vi "PV Miscellaneous.vi"(8 "error in (no error)":errorcluster, 9 "PV Miscellaneous - Cluster":T1={"Parameter"=0, "Parameter\nread only<->describe"=FALSE, "off<->on   "=TRUE, "Unit adress"=1, "Configuration AO1 (old version)"=0, "Contens of service\nline; # of the 2nd\n parameter"=795, "Configuration DO1 (old version)"=0} {"Configuration DO1 (old version)" items=[" switchpoint attained", " no error", " error", " warning", " error and/or warning", " set speed attained", " pump is on", " accelerates", " decelerater", " always off", " always on", " access request remote"]; "Contens of service\nline; # of the 2nd\n parameter" min=0 max=999 step=1; "Configuration AO1 (old version)" items=[" speed", " power", " current", " lowest value", " highest value"]; "Unit adress" min=1 max=255 step=1; "Parameter" items=[" Preselection brake", " Configuration DO1 (old version)", " Remote operations mode", " Configuration output K4 (old version)", " Configuration AO1 (old version)", " Actual error code (read only)", " Software version electronic drive unit  (read only)", " Software version display and control unit  (read only)", " Parameter set", " Contens of service line (TCM 1601 only)", " Unit adress", " Unit type electronic drive unit", " Error acknowledgement (write only)", " Keyboard interlock (008)", " Seal gas enable (050)"]}, 10 "Adress of unit":u16=1 max=999 step=1, 11 "VISA session":refnum<visa-resource-name>) -> (0 "error out":errorcluster, 2 "response (data)":string, 3 "dup VISA session":refnum<visa-resource-name>)   [LabVIEW 2016, in "Pfeiffer Vacuum.lvlib"]
doc: "There are 15 parameters available, only one of which can be enabled at a time. \n\nPreselection brake (default) (013)\nConfiguration DO1 (024)\n(old version - new in PV Config A D input output)\nRemote operations mode (028)\nConfiguration output K4 (032)\n (old version - new in PV Config A D input output)\nConfiguration AO1 (055)\n (old version - new in PV Config A D input output)\nActual error code (read only) (303)\nSoftware version electronic drive unit (read only) (312)\nSoftware version display and control unit (read only) (351)\nParameter set (794)\nContens of service line (TCM 1601 only) (795)\nUnit adress (797)\nUnit type electronic drive unit (349)\nError acknowledgement (write only) (009)\nKeyboard interlock (008)\nSeal gas enable (050)\n\nNote: Any settings for an parameter that is not selected will be ignored. If a value is out of range, it will be changed to either the upper or the lower limit of the range."
uses:
  Pfeiffer Vacuum.lvlib
  PV Miscellaneous - Cluster.ctl
panel:
  # "Preselection brake             :  \n Remote operations mode  : \n Configuration output K4    : \n Parameter set                      :\n Seal gas enable                   :\n Keyboard interlock            :"
  # "<--------------\n  off\n  stand. operations \n  heat/TMS\n  basic  \n  off\n  off"
  # "----------->          \non \nremote priority \nPWM-signal \n extended \non \non"
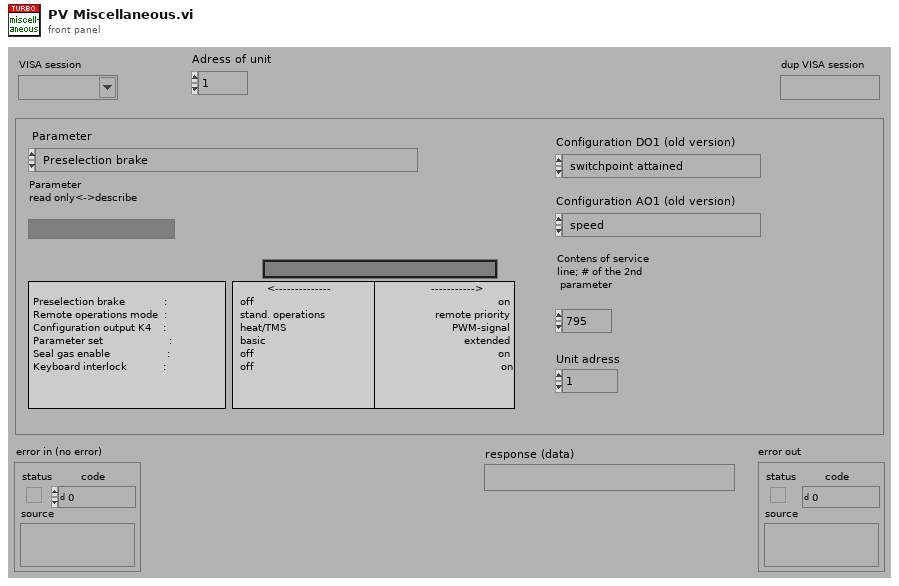
[diagram p1: front panel]
types:
  T1 = typedef "Pfeiffer Vacuum.lvlib/PV Miscellaneous - Cluster.ctl" = cluster{"Parameter":u16, "Parameter\nread only<->describe":bool, "off<->on   ":bool, "Unit adress":i16, "Configuration AO1 (old version)":u16, "Contens of service\nline; # of the 2nd\n parameter":i16, "Configuration DO1 (old version)":u16}
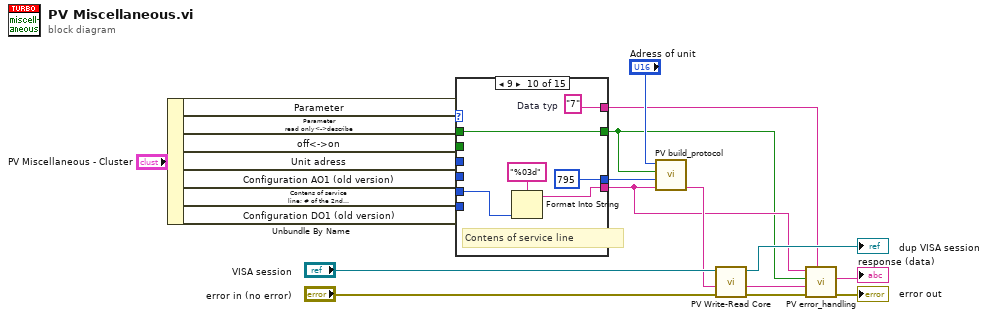
[diagram p0: block diagram]
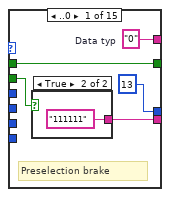
[diagram p2: hidden frame]
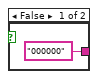
[diagram p3: hidden frame]
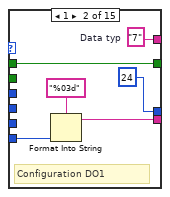
[diagram p4: hidden frame]
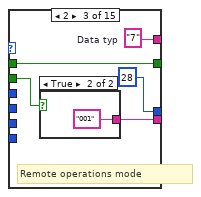
[diagram p5: hidden frame]
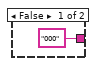
[diagram p6: hidden frame]
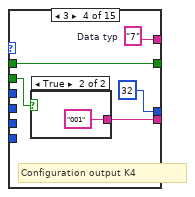
[diagram p7: hidden frame]
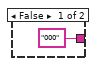
[diagram p8: hidden frame]
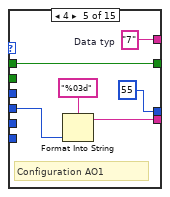
[diagram p9: hidden frame]
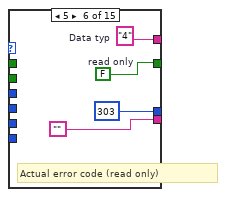
[diagram p10: hidden frame]
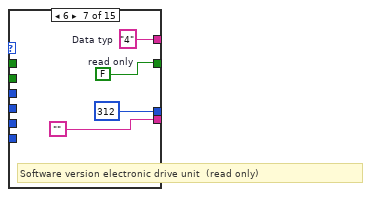
[diagram p11: hidden frame]
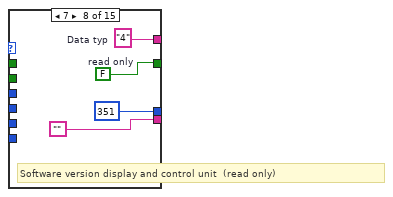
[diagram p12: hidden frame]
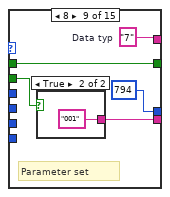
[diagram p13: hidden frame]
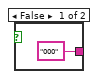
[diagram p14: hidden frame]
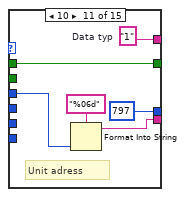
[diagram p15: hidden frame]
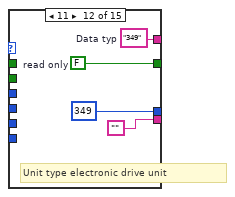
[diagram p16: hidden frame]
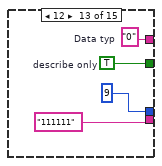
[diagram p17: hidden frame]
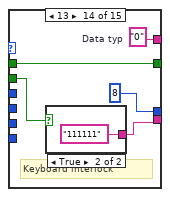
[diagram p18: hidden frame]
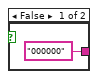
[diagram p19: hidden frame]
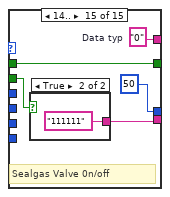
[diagram p20: hidden frame]
diagram:
  n1 = Unbundle By Name("PV Miscellaneous - Cluster") -> ("Parameter"=w18:u16, "Parameter\nread only<->describe"=w17:bool, "off<->on"=w15:bool, "Unit adress"=w14:i16, "Configuration AO1 (old version)"=w13:u16, "Contens of service\nline; # of the 2nd\n parameter"=w12:i16, "Configuration DO1 (old version)"=w1:u16)
  n2 = case shown="9" w18 {
    tunnel: [u16 13 ("Parameter-number") u16 24 ("Parameter-number") u16 28 ("Parameter-number") u16 32 ("Parameter-number") u16 55 ("Parameter-number") u16 303 ("Parameter-number") u16 312 ("Parameter-number") u16 351 ("Parameter-number") u16 794 ("Parameter-number") u16 795 ("Parameter-number") u16 797 ("Parameter-number") u16 349 ("Parameter-number") u16 9 ("Parameter-number") u16 8 ("Parameter-number") u16 50 ("Parameter-number")] -> w20
    tunnel: [w25 w30 w38 w45 w52 "" "" "" w70 w78 w84 "" "111111" ("Data") w94 w102] -> w4
    tunnel: [w24 w33 w37 w44 w53 w57 w61 w65 w69 w76 w82 w89 w93 w96 w104] -> w3
    tunnel: w17 -> [w24 w33 w37 w44 w53 _ _ _ w69 w76 w82 _ _ w96 w104]
    tunnel: w15 -> [w23 _ w36 w43 _ _ _ _ w68 _ _ _ _ w95 w103]
    tunnel: w14 -> [_ _ _ _ _ _ _ _ _ _ w81 _ _ _ _]
    tunnel: w13 -> [_ _ _ _ w51 _ _ _ _ _ _ _ _ _ _]
    tunnel: w12 -> [_ _ _ _ _ _ _ _ _ w75 _ _ _ _ _]
    tunnel: [w22 w32 w35 w42 w49 w55 w59 w63 w67 w74 w80 w86 w90 w97 w105] -> w5
    tunnel: w1 -> [_ w31 _ _ _ _ _ _ _ _ _ _ _ _ _]
    frame ..0 {
      w22 = "0"  # Data typ
      # "Preselection brake"
      n3 = case shown="True" w23 {
        tunnel: ["000000" ("Data") "111111" ("Data")] -> w25
        frame False {
        }
        frame True {
        }
      }
    }
    frame 1 {
      w32 = "7"  # Data typ
      # "Configuration DO1"
      n4 = Format Into String(format string="%03d" ("Format-String"), w31) -> (resulting string=w30:string)  [unwired: 2 in, 1 out]
    }
    frame 2 {
      w35 = "7"  # Data typ
      # "Remote operations mode"
      n5 = case shown="True" w36 {
        tunnel: ["000" ("Data") "001" ("Data")] -> w38
        frame False {
        }
        frame True {
        }
      }
    }
    frame 3 {
      w42 = "7"  # Data typ
      # "Configuration output K4"
      n6 = case shown="True" w43 {
        tunnel: ["000" ("Data") "001" ("Data")] -> w45
        frame False {
        }
        frame True {
        }
      }
    }
    frame 4 {
      w49 = "7"  # Data typ
      # "Configuration AO1"
      n7 = Format Into String(format string="%03d" ("Format-String"), w51) -> (resulting string=w52:string)  [unwired: 2 in, 1 out]
    }
    frame 5 {
      w55 = "4"  # Data typ
      w57 = FALSE  # read only
      # "Actual error code (read only)"
    }
    frame 6 {
      w59 = "4"  # Data typ
      w61 = FALSE  # read only
      # "Software version electronic drive unit  (read only)"
    }
    frame 7 {
      w63 = "4"  # Data typ
      w65 = FALSE  # read only
      # "Software version display and control unit  (read only)"
    }
    frame 8 {
      w67 = "7"  # Data typ
      # "Parameter set"
      n8 = case shown="True" w68 {
        tunnel: ["000" ("Data") "001" ("Data")] -> w70
        frame False {
        }
        frame True {
        }
      }
    }
    frame 9 {
      w74 = "7"  # Data typ
      # "Contens of service line"
      n9 = Format Into String(format string="%03d" ("Format-String"), w75) -> (resulting string=w78:string)  [unwired: 2 in, 1 out]
    }
    frame 10 {
      w80 = "1"  # Data typ
      # "Unit adress"
      n10 = Format Into String(format string="%06d" ("Format-String"), w81) -> (resulting string=w84:string)  [unwired: 2 in, 1 out]
    }
    frame 11 {
      w86 = "349"  # Data typ
      w89 = FALSE  # read only
      # "Unit type electronic drive unit"
    }
    frame 12 {
      w90 = "0"  # Data typ
      w93 = TRUE  # describe only
    }
    frame 13 {
      w97 = "0"  # Data typ
      # "Keyboard interlock"
      n11 = case shown="True" w95 {
        tunnel: ["000000" ("Data") "111111" ("Data")] -> w94
        frame False {
        }
        frame True {
        }
      }
    }
    frame 14.. {
      w105 = "0"  # Data typ
      # "Sealgas Valve 0n/off"
      n12 = case shown="True" w103 {
        tunnel: ["000000" ("Data") "111111" ("Data")] -> w102
        frame False {
        }
        frame True {
        }
      }
    }
  }
  n13 = call "PV build_protocol.vi"("Data"=w4, "Parameter-number"=w20, "parameter\nread<->describe"=w3, "Adress"="Adress of unit") -> ("output"=w9:string)  [unwired: 3 in]
  n14 = call "PV Write-Read Core.vi"("error in"="error in (no error)", "Write data in"=w9, "VISA session"="VISA session") -> ("error out"=w6:errorcluster, "response (data) out"=w7:string, "dup VISA session"=→"dup VISA session":refnum<visa-resource-name>)  [unwired: 2 in]
  n15 = call "PV error_handling.vi"("Data Typ in"=w5, "error in"=w6, "response (data) in"=w7, "Parameter\nread only<->describe"=w3, "data in"=w4) -> ("error out"=→"error out":errorcluster, "Data out"=→"response (data)":string)  [unwired: 4 in, 1 out]
